vi "Run RT Sequence Numeric Limit Test.vi"(0 "Sequence Context":refnum<k7>, 1 "Sequence File Path":path, 5 "ParamNames":string[](array[string]), 7 "ParamValues":string[](array[string]), 9 "ParamTypes":string[](array[string]), 10 "NumericDataType":string, 11 "Target (\"\": Auto-assign)":string, 13 "Timeout (ms)":dbl=10000.0, 14 "Gateway IP Address":string) -> (4 "Report Text":string, 8 "Numeric":dbl, 15 "error out":errorcluster)   [LabVIEW 2015]
doc: "Executes a single pass of a real-time sequence giving the defined parameter names, values, and types. Outputs a pass/fail value if the numeric return value is within the specified lower and upper limits."
uses:
  <vilib>/NI Veristand/Execution/SequenceExecutionInterface/Sequence Execution State.ctl
  NationalInstruments.VeriStand.DataTypes
  <vilib>/NI Veristand/Execution/SequenceExecutionInterface/NI_VS Sequence Execution Interface.lvlib
  RTSequenceVIs.lvlib
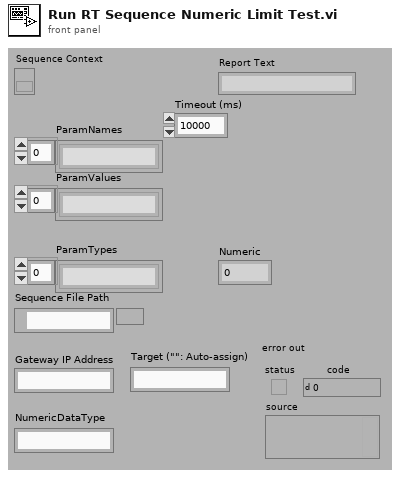
[diagram p1: front panel]
types:
  T1 = typedef "NI_VS Sequence Execution Interface.lvlib/Sequence Input Assignment Ref.ctl" = refnum<k24>
  T2 = typedef "NI_VS Sequence Execution Interface.lvlib/Sequence Call Ref.ctl" = refnum<k24>
  T3 = typedef "NI_VS Sequence Execution Interface.lvlib/Stimulus Profile Session Ref.ctl" = refnum<k24>
  T4 = typedef "TestStand - Status Monitor.ctl" = cluster{"Sequence Context":refnum<k7>, "Execution":refnum<k7>, "Termination Monitor":refnum<k7>}
  T5 = typedef "NI_VS Sequence Execution Interface.lvlib/Sequence Execution State.ctl" = enum16{"Idle", "Running", "SingleStepping", "Paused", "Stopped"}
  T6 = typedef "NI_VS Sequence Execution Interface.lvlib/Data Value Ref.ctl" = refnum<k24>
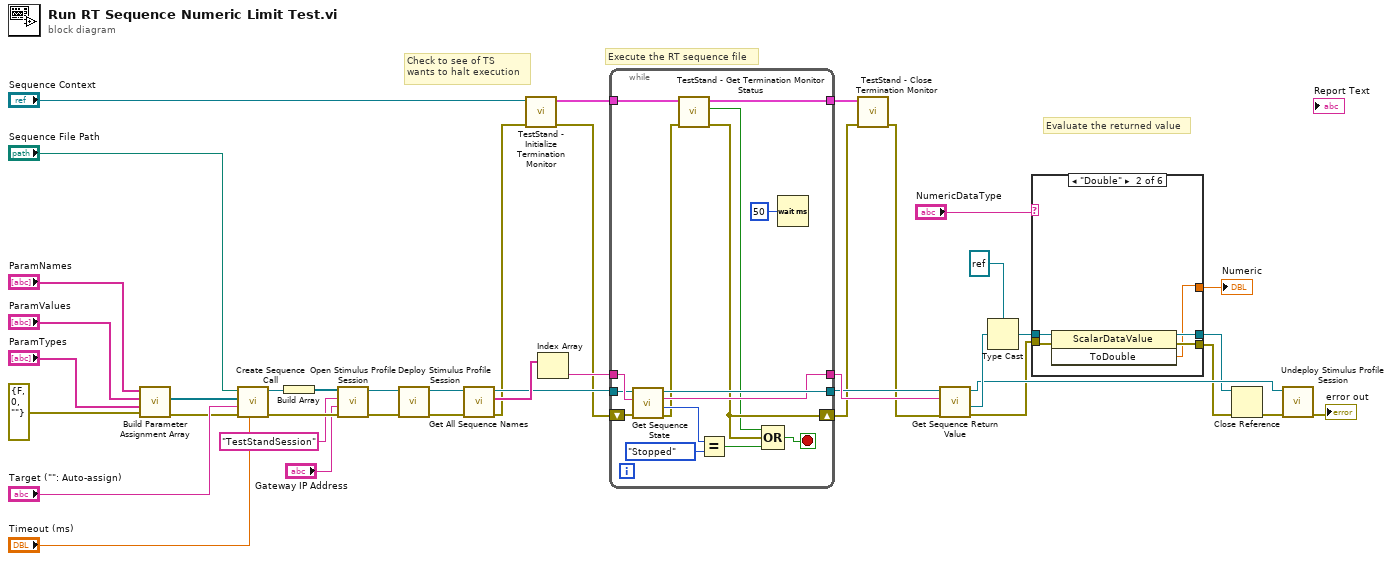
[diagram p0: block diagram]
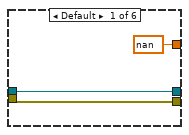
[diagram p2: hidden frame]
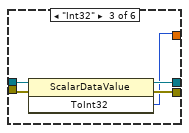
[diagram p3: hidden frame]
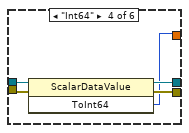
[diagram p4: hidden frame]
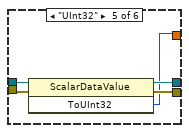
[diagram p5: hidden frame]
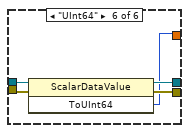
[diagram p6: hidden frame]
diagram:
  # "Check to see of TS\nwants to halt execution"
  # "Evaluate the returned value"
  # "Execute the RT sequence file"
  n1 = call "Build Parameter Assignment Array.vi"("error in (no error)"=errorcluster {"status"=FALSE, "code"=0, "source"=""}, "ParamTypes"="ParamTypes", "ParamValues"="ParamValues", "ParamNames"="ParamNames") -> ("error out"=w6:errorcluster, "Sequence Parameter Assignment refs"=w5:T1[])  [unwired: 6 in]
  n2 = call <vilib>:"Create Sequence Call.vi"("Timeout ms (10000)"="Timeout (ms)", "error in (no error)"=w6, "Target (\"\": Auto-assign)"="Target (\"\": Auto-assign)", "Parameter Assignments"=w5, "Sequence File Path"="Sequence File Path") -> ("error out"=w40:errorcluster, "Sequence Call Ref"=w34:T2)  [unwired: 5 in]
  n3 = Build Array(w34) -> (w38:T2[])
  n4 = call <vilib>:"Open Stimulus Profile Session.vi"("error in (no error)"=w40, "Gateway IP Address (\"\": localhost)"="Gateway IP Address", "Session Name"="TestStandSession", "Sequence Calls"=w38) -> ("error out"=w36:errorcluster, "Session Ref"=w37:T3)  [unwired: 6 in]
  n5 = call <vilib>:"Deploy Stimulus Profile Session.vi"("error in (no error)"=w36, "Session Ref in"=w37) -> ("error out"=w33:errorcluster, "Session Ref out"=w32:T3)  [unwired: 7 in, 1 out]
  n6 = call <vilib>:"Get All Sequence Names.vi"("error in (no error)"=w33, "Session Ref in"=w32) -> ("error out"=w14:errorcluster, "Sequence Names out"=w31:string[], "Session Ref out"=w29:T3)  [unwired: 7 in]
  n7 = call <vilib>:"TestStand - Initialize Termination Monitor.vi"("error in (no error)"=w14, "Sequence Context In"="Sequence Context") -> ("error out"=w13:errorcluster, "Status Monitor Out"=w12:T4)  [unwired: 8 in]
  n8 = Index Array(array=w31) -> (element=w30:string)  [unwired: 1 in]
  n9 = while {
    tunnel: w30 -> [w56]
    tunnel: w29 -> [w55]
    shift-right: [w44] -> w10
    shift-left: w13 -> [w54]
    tunnel: [w49] -> w24
    tunnel: [w47] -> w28
    tunnel: w12 -> [w46]
    tunnel: [w42] -> w11
    stop <- w50 stop-if-true
    n10 = call <vilib>:"Get Sequence State.vi"("error in (no error)"=w54, "Sequence Name"=w56, "Session Ref in"=w55) -> ("error out"=w45:errorcluster, "State"=w53:T5, "Sequence Name out"=w47:string, "Session Ref out"=w49:T3)  [unwired: 5 in]
    n11 = call <vilib>:"TestStand - Get Termination Monitor Status.vi"("error in (no error)"=w45, "Status Monitor In"=w46) -> ("error out"=w44:errorcluster, "Terminating or Aborting"=w43:bool, "Status Monitor Out"=w42:T4)  [unwired: 7 in]
    n12 = Equal?(x=w53, y=Sequence_Execution_State."Stopped" ("State")) -> (x = y?=w51:bool)
    n13 = Compound Arithmetic op=OR(w43, w44, w51) -> (w50:bool)
    n14 = Wait (ms)(milliseconds to wait=u32 50 ("millisecond multiple")) -> ()  [unwired: 1 out]
  }
  n15 = call <vilib>:"TestStand - Close Termination Monitor.vi"("error in (no error)"=w10, "Status Monitor In"=w11) -> ("error out"=w9:errorcluster)  [unwired: 9 in]
  n16 = call <vilib>:"Get Sequence Return Value.vi"("error in (no error)"=w9, "Sequence Name"=w28, "Session Ref in"=w24) -> ("error out"=w22:errorcluster, "Data Value Ref"=w27:T6, "Session Ref out"=w23:T3)  [unwired: 5 in, 1 out]
  n17 = Type Cast(type=refnum<k24> refnum ("Node"), x=w27) -> (*(type *) &x=w25:refnum<k24>)
  n18 = case shown="\"Double\"" "NumericDataType" {
    tunnel: w25 -> [w58 w64 w69 w74 w79 w84]
    tunnel: w22 -> [w59 w63 w68 w73 w78 w83]
    tunnel: [w59 w62 w67 w72 w77 w82] -> w21
    tunnel: [w58 w61 w66 w71 w76 w81] -> w19
    tunnel: [nan ("ToDouble") w60 w65 w70 w75 w80] -> w17
    frame Default {
    }
    frame "Double" {
      n19 = invoke class="ScalarDataValue" method="ToDouble"(reference=w64, error in=w63) -> (reference out=w61:refnum<k24>, error out=w62:errorcluster, "ToDouble"=w60:dbl)  [unwired: 1 in]
    }
    frame "Int32" {
      n20 = invoke class="ScalarDataValue" method="ToInt32"(reference=w69, error in=w68) -> (reference out=w66:refnum<k24>, error out=w67:errorcluster, "ToInt32"=w65:i32)  [unwired: 1 in]
    }
    frame "Int64" {
      n21 = invoke class="ScalarDataValue" method="ToInt64"(reference=w74, error in=w73) -> (reference out=w71:refnum<k24>, error out=w72:errorcluster, "ToInt64"=w70:i64)  [unwired: 1 in]
    }
    frame "UInt32" {
      n22 = invoke class="ScalarDataValue" method="ToUInt32"(reference=w79, error in=w78) -> (reference out=w76:refnum<k24>, error out=w77:errorcluster, "ToUInt32"=w75:u32)  [unwired: 1 in]
    }
    frame "UInt64" {
      n23 = invoke class="ScalarDataValue" method="ToUInt64"(reference=w84, error in=w83) -> (reference out=w81:refnum<k24>, error out=w82:errorcluster, "ToUInt64"=w80:u64)  [unwired: 1 in]
    }
  }
  "Numeric" <- w17
  n24 = Close Reference(reference=w19, error in (no error)=w21) -> (error out=w20:errorcluster)
  n25 = call <vilib>:"Undeploy Stimulus Profile Session.vi"("error in (no error)"=w20, "Session Ref in"=w23) -> ("error out"=→"error out":errorcluster)  [unwired: 8 in, 1 out]
